vi "updater.vi"() -> ()   [LabVIEW 2014]
uses:
  <vilib>/Utility/sysdir.llb/System Directory Type.ctl
  subVI/version.vi
  <vilib>/Utility/config.llb/Read Key (String).vi
  <vilib>/FTP/NI_FTP.lvlib
  <vilib>/Utility/config.llb/NI_LVConfig.lvlib
panel:
  out "슬라이드":u8(slide) scale=1.0..3.0
  out "정보출력":string="업데이트 정보를 확인합니다."
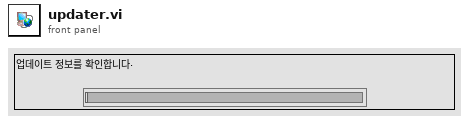
[diagram p1: front panel]
types:
  T1 = typedef "NI_FTP.lvlib/FTP Session.ctl" = refnum<k5>
  T2 = typedef "System Directory Type.ctl" = i32
  T3 = typedef "NI_LVConfig.lvlib/Config Data RefNum.ctl" = refnum<k1>
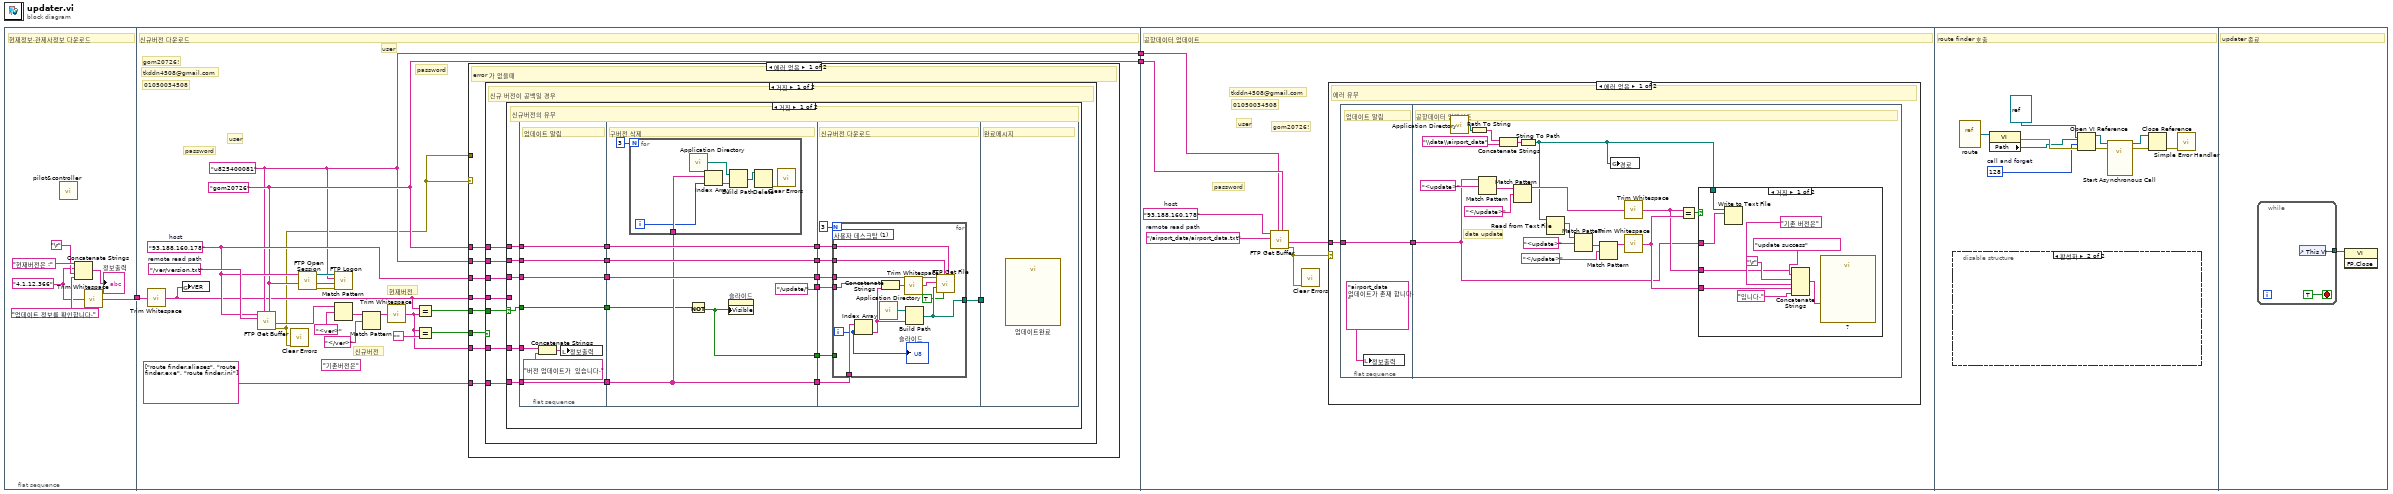
[diagram p0: block diagram]
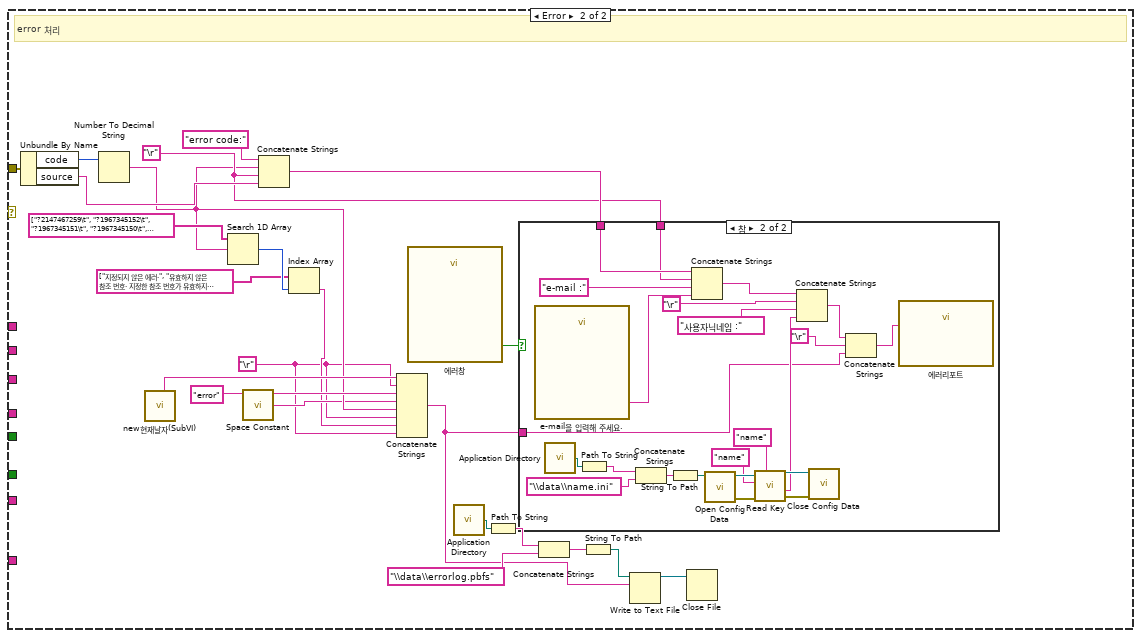
[diagram p4: hidden frame]
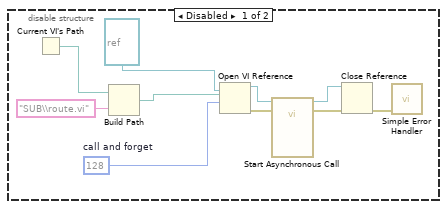
[diagram p8: hidden frame]
diagram:
  n1 = flat-sequence {
    tunnel: [w5] -> w1
    tunnel: [w17] -> w3
    tunnel: [w18] -> w2
    tunnel: w1 -> [w16]
    tunnel: w3 -> [w151]
    tunnel: w2 -> [w152]
    frame #0 {
      w4 = "4.1.12.366"
      # "현재정보,관제사정보 다운로드"
      n2 = call "pilot&controller.vi"() -> ()  [unwired: 11 in, 1 out]
      n3 = Concatenate Strings("현재버전은 :", w4, "\r", "업데이트 정보를 확인합니다." ("정보출력")) -> (→"정보출력":string)
      n4 = call <vilib>:"Trim Whitespace.vi"("string"=w4) -> ("trimmed string"=w5:string)  [unwired: 1 in]
    }
    frame #1 {
      (unwired) "기존버전은" ("문자열")
      w18 = "gom20726"
      w17 = "u825400081"
      w26 = "/ver/version.txt"  # remote read path
      w19 = "93.188.160.178"  # host
      # "신규버전"
      # "현재버전"
      # "password"
      # "user"
      # "gom20726!"
      # "01050034508"
      # "tkddn4508@gmail.com"
      # "user"
      # "password"
      # "신규버전 다운로드"
      n5 = call <vilib>:"Trim Whitespace.vi"("string"=w16) -> ("trimmed string"=w13:string)  [unwired: 1 in]
      n6 = global write "version.vi" "VER"(w13) -> ()
      n7 = call <vilib>:"FTP Get Buffer.vi"("password"=w18, "user"=w17, "remote path"=w26, "host"=w19) -> ("error out"=w12:errorcluster, "data"=w24:string)  [unwired: 5 in, 1 out]
      n8 = call <vilib>:"Clear Errors.vi"("error in (no error)"=w12) -> ()  [unwired: 5 in, 2 out]
      n9 = call <vilib>:"FTP Open Session.vi"("address"=w19) -> ("error out"=w28:errorcluster, "ftp session"=w27:T1)  [unwired: 7 in, 2 out]
      n10 = call <vilib>:"FTP Logon.vi"("error in (no error)"=w28, "password"=w18, "user"=w17, "ftp session"=w27) -> ()  [unwired: 4 in, 4 out]
      n11 = Match Pattern(string=w24, regular expression="<ver>" ("정규식")) -> (after substring=w23:string)  [unwired: 1 in, 3 out]
      n12 = Match Pattern(string=w23, regular expression="</ver>" ("정규식")) -> (before substring=w21:string)  [unwired: 1 in, 3 out]
      n13 = call <vilib>:"Trim Whitespace.vi"("string"=w21) -> ("trimmed string"=w14:string)  [unwired: 1 in]
      n14 = Equal?(x=w13, y=w14) -> (x = y?=w10:bool)
      n15 = Equal?(x=w14, y="") -> (x = y?=w11:bool)
      n16 = case shown="에러 없음" w12 {
        tunnel: w19 -> [w36 _]
        tunnel: w17 -> [w35 _]
        tunnel: w18 -> [w34 _]
        tunnel: string[] ["route finder.aliases", "route finder.exe", "route finder.ini"] -> [w33 _]
        tunnel: w12 -> [_ w125]
        tunnel: w13 -> [w32 _]
        tunnel: w14 -> [w31 _]
        tunnel: w11 -> [w30 _]
        tunnel: w10 -> [w29 _]
        frame No Error {
          # "error 가 없을때"
          n17 = case shown="거짓" w30 {
            tunnel: w36 -> [w43 _]
            tunnel: w35 -> [w42 _]
            tunnel: w34 -> [w41 _]
            tunnel: w33 -> [w40 _]
            tunnel: w32 -> [w39 _]
            tunnel: w31 -> [w38 _]
            tunnel: w29 -> [w37 _]
            frame False {
              # "신규 버전이 공백일 경우"
              n18 = case shown="거짓" w37 {
                selector: w37 -> [w45 _]
                tunnel: w43 -> [w61 _]
                tunnel: w42 -> [w60 _]
                tunnel: w41 -> [w59 _]
                tunnel: w40 -> [w58 _]
                tunnel: w39 -> [_ _]
                tunnel: w38 -> [w47 _]
                frame False {
                  # "신규버전의 유무"
                  n19 = flat-sequence {
                    tunnel: w58 -> [w66]
                    tunnel: w59 -> [w67]
                    tunnel: w60 -> [w68]
                    tunnel: w61 -> [w69]
                    tunnel: [w69] -> w51
                    tunnel: [w68] -> w50
                    tunnel: [w67] -> w49
                    tunnel: [w66] -> w48
                    tunnel: w47 -> [w63]
                    tunnel: [w62] -> w46
                    tunnel: w45 -> [w62]
                    tunnel: [w77] -> w57
                    tunnel: [w76] -> w56
                    tunnel: [w75] -> w55
                    tunnel: ["/update/" ("remote path")] -> w54
                    tunnel: [w73] -> w53
                    tunnel: w51 -> [w77]
                    tunnel: w50 -> [w76]
                    tunnel: w49 -> [w75]
                    tunnel: w48 -> [w73]
                    tunnel: w46 -> [w71]
                    tunnel: [w70] -> w44
                    tunnel: w57 -> [w91]
                    tunnel: w56 -> [w90]
                    tunnel: w55 -> [w89]
                    tunnel: w54 -> [w88]
                    tunnel: w53 -> [w86]
                    tunnel: [w85] -> w52
                    tunnel: w44 -> [w84]
                    tunnel: w52 -> [_]
                    frame #0 {
                      # "업데이트 알림"
                      n20 = Concatenate Strings(w63, "버전 업데이트가  있습니다." ("문자열")) -> (w65:string)
                      n21 = local write "정보출력"(w65) -> ()
                    }
                    frame #1 {
                      # "구버전 삭제"
                      n22 = for {
                        N: 3 -> [_]
                        tunnel: w73 -> [w79]
                        i -> [w78]
                        n23 = call <vilib>:"Application Directory.vi"() -> ("Application Directory"=w83:path)
                        n24 = Index Array(array=w79, index=w78) -> (element=w82:string)
                        n25 = Build Path(base path=w83, name or relative path=w82) -> (appended path=w81:path)
                        n26 = Delete(path (use dialog)=w81) -> (error out=w80:errorcluster)  [unwired: 4 in, 2 out]
                        n27 = call <vilib>:"Clear Errors.vi"("error in (no error)"=w80) -> ()  [unwired: 5 in, 2 out]
                      }
                      n28 = Not(x=w71) -> (.not. x?=w70:bool)
                      n29 = property on="슬라이드" class="Slide (엄격한)"("Visible"=w70) -> ()  [unwired: 2 in, 2 out]
                    }
                    frame #2 {
                      # "신규버전 다운로드"
                      n30 = for {
                        N: 3 -> [_]
                        tunnel: w91 -> [w103]
                        tunnel: w90 -> [w102]
                        tunnel: w89 -> [w101]
                        tunnel: w88 -> [w100]
                        tunnel: w86 -> [w97]
                        tunnel: [w96] -> w85
                        tunnel: w84 -> [_]
                        i -> [w92]
                        (unwired) T2 1 items=["사용자 홈"=0, "사용자 데스크탑"=1, "사용자 문서"=2, "사용자 어플리케이션 데이터"=3, "사용자 환경"=4, "사용자 임시"=5, "퍼블릭 문서"=6, "퍼블릭 어플리케이션 데이터"=7, "퍼블릭 환경"=8, "퍼블릭 캐시"=13, "시스템 코어 라이브러리"=9, "시스템 설치된 라이브러리"=10, "어플리케이션 파일"=11, "부팅 볼륨 루트"=12] ("system directory type")
                        n31 = Index Array(array=w97, index=w92) -> (element=w95:string)
                        n32 = call <vilib>:"Application Directory.vi"() -> ("Application Directory"=w93:path)
                        n33 = Concatenate Strings(w100, w95) -> (w99:string)
                        n34 = call <vilib>:"Trim Whitespace.vi"("string"=w99) -> ("trimmed string"=w98:string)  [unwired: 1 in]
                        n35 = Build Path(base path=w93, name or relative path=w95) -> (appended path=w96:path)
                        n36 = call <vilib>:"FTP Get File.vi"("password"=w101, "binary (F)"=TRUE, "user"=w102, "local path"=w96, "remote path"=w98, "host"=w103) -> ()  [unwired: 4 in, 2 out]
                        "슬라이드" <- w92
                      }
                    }
                    frame #3 {
                      # "완료메시지"
                      n37 = call "업데이트완료"() -> ()  [unwired: 10 in, 2 out]
                    }
                  }
                }
                frame True {
                }
              }
            }
            frame True {
            }
          }
        }
        frame Error {
          w105 = "\r"
          w120 = "\r"
          # "error 처리"
          n38 = Unbundle By Name(w125) -> ("code"=w124:i32, "source"=w122:string)
          n39 = Number To Decimal String(number=w124) -> (decimal integer string=w108:string)  [unwired: 1 in]
          n40 = call "new현재날자(SubVI).vi"() -> ("날짜/시간 문자열"=w110:string)  [unwired: 5 in, 6 out]
          n41 = Search 1D Array(1D array=string[] ["?2147467259\t", "?1967345152\t", "?1967345151\t", "?1967345150\t", "?1967345149\t", "?1967345148\t", "?1967345147\t", "?375012\t", "?375011\t", "?375010\t", "?375009\t", "?375008\t", "?375007\t", "?375005\t", "?375004\t", "?375003\t", "?375002\t", "?375001\t", "?375000\t", "?120000", "?4850\t", "?4824\t", "?4820\t", "?4803\t", "?4407\t", "?4406\t", "?4404\t", "?4403\t", "?4402\t", "?4401\t", "?4400\t", "?2584\t", "?2580\t", "1\t", "2\t", "4\t", "5\t", "6\t", "7\t", "8\t", "9\t", "10\t", "11\t", "12\t", "13\t", "14\t", "15\t", "16\t", "17\t", "18\t", "19\t", "20\t", "21\t", "22\t", "23\t", "24\t", "25\t", "26\t", "27\t", "28", "29\t", "30\t", "31\t", "32\t", "33\t", "34\t", "35\t", "36\t", "37\t", "38\t", "39\t", "40\t", "41\t", "42\t", "43\t", "44\t", "45\t", "46\t", "47\t", "48\t", "49\t", "50\t", "51", "52\t", "67\t", "68\t", "69\t", "70\t", "71\t", "72\t", "73\t", "74\t", "75\t", "81\t", "82\t", "83\t", "84\t", "85\t", "87\t", "88\t", "89\t", "90\t", "91\t", "97\t", "98\t", "99\t", "100\t", "116\t", "117\t", "118\t", "122\t", "123\t", "124\t", "125\t", "1000\t", "1001\t", "1002\t", "1003\t", "1004\t", "1005\t", "1006\t", "1007\t", "1008\t", "1009\t", "1010\t", "1011\t", "1012\t", "1013\t", "1014\t", "1015\t", "1016\t", "1017\t", "1018\t", "1019\t", "1022\t", "1023\t", "1024\t", "1025\t", "1026\t", "1027\t", "1028\t", "1029\t", "1030\t", "1031\t", "1032\t", "1033\t", "1034\t", "1035\t", "1036\t", "1037\t", "1038", "1039\t", "1040\t", "1041\t", "1042\t", "1043\t", "1044\t", "1045\t", "1051\t", "1052\t", "1054\t", "1055\t", "1056\t", "1057\t", "1058\t", "1059\t", "1060\t", "1061", "1062\t", "1063\t", "1066\t", "1067\t", "1068\t", "1069\t", "1070\t", "1071\t", "1072\t", "1073\t", "1074\t", "1075\t", "1076\t", "1077\t", "1082\t", "1086\t", "1087\t", "1088\t", "1089\t", "1090\t", "1091\t", "1094\t", "1095\t", "1096\t", "1097\t", "1098\t", "1100\t", "1102\t", "1103\t", "1104\t", "1105\t", "1106\t", "1107\t", "1108\t", "1109\t", "1110\t", "1111\t", "1122\t", "1123\t", "1124\t", "1125\t", "1126\t", "1127\t", "1128\t", "1129\t", "1130\t", "1131\t", "1135\t", "1136\t", "1137\t", "1138\t", "1144\t", "1145\t", "1146\t", "1147\t", "1148\t", "1149\t", "1150\t", "1151\t", "1156\t", "1157\t", "1174\t", "1175\t", "1176\t", "1177\t", "1186\t", "1187\t", "1188\t", "1190\t", "1191\t", "1192\t", "1193\t", "1194\t", "1196\t", "1197\t", "1198\t", "1301\t", "1303\t", "1304\t", "1305\t", "1306\t", "1307\t", "1308\t", "1309\t", "1310\t", "1311\t", "1312\t", "1313\t", "1314\t", "1315\t", "1319\t", "1320\t", "1321\t", "1322\t", "1357\t", "1358\t", "1359\t", "1360\t", "1361\t", "1362\t", "1363\t", "1364\t", "1365\t", "1366\t", "1370\t", "1376\t", "1377\t", "1378\t", "1380\t", "1381\t", "1384\t", "1385\t", "1388\t", "1389\t", "1390\t", "1396\t", "1397\t", "1398\t", "1399\t", "1430\t", "1432\t", "1434\t", "1436\t", "1438\t", "1439", "1440\t", "1443", "1444", "1445\t", "1447\t", "1449\t", "1450\t", "1451\t", "1452\t", "1453\t", "1454\t", "1455\t", "1468\t", "1469\t", "1470\t", "1483\t", "1484\t", "1485\t", "1488\t", "1489\t", "1490\t", "1491\t", "1492\t", "1493\t", "1497\t", "1498\t", "1499\t", "1500\t", "1502\t", "1503\t", "1504\t", "1517\t", "1523\t", "1524\t", "1526\t", "1529\t", "1532\t", "1533\t", "1534\t", "1535\t", "1544\t", "1545\t", "1546\t", "1548\t", "1550\t", "1553\t", "1554\t", "1556\t", "1557\t", "1558\t", "1564\t", "1571\t", "1573\t", "1574\t", "1579\t", "1580\t", "1581\t", "1584\t", "1586\t", "1587\t", "1588\t", "1590\t", "1595\t", "1596\t", "1597\t", "1599\t", "1603\t", "1604\t", "1611\t", "1616\t", "1617\t", "1619\t", "1620\t", "1621\t", "1622\t", "1623\t", "1624\t", "1627\t", "1628\t", "1629\t", "1630\t", "1632\t", "4800\t", "4801\t", "4802\t", "4803\t", "4804\t", "4805\t", "4806\t", "4810\t", "4811\t", "4820\t", "4821\t", "4822\t", "4823\t", "56000\t", "56001\t", "56002\t", "56003\t", "56004", "56005\t", "56006\t", "66464"] ("String Data"), element=w108) -> (index of element=w113:i32)  [unwired: 1 in]
          n42 = call <vilib>:"Space Constant.vi"() -> ("String"=w107:string)
          n43 = Concatenate Strings("error code:" ("문자열"), w108, w120, w122) -> (w121:string)
          n44 = Index Array(array=string[] ["지정되지 않은 에러.", "유효하지 않은 참조 번호. 지정한 참조 번호가 유효하지 않습니다.", "유효하지 않은 프로퍼티 코드. 지정한 프로퍼티 코드가 이 참조 번호에는 유효하지 않습니다.", "유효하지 않은 특권 ID. 지정한 특권 ID가 범위를 벗어납니다.", "유효하지 않은 접근 타입. 지정한 접근 타입이 유효하지 않습니다.", "유효하지 않은 인수. 지정한 인수 중 하나가 유효하지 않습니다.", "발견되지 않은 입력. 요청하신 입력을 찾을 수 없습니다.", "JSON 숫자값이 LabVIEW 숫자형 타입의 범위를 벗어납니다.", "LabVIEW가 무한대 또는 무한대 부동소수 값을 읽거나 쓰는데 실패했습니다. 무한대 값에 대한 지원을 허용하려면 LabVIEW JSON을 활성화해야 합니다.", "LabVIEW가 NaN 부동소수 값을 읽거나 쓰는데 실패했습니다. NaN 값에 대한 지원을 허용하려면 LabVIEW JSON을 활성화해야 합니다.", "JSON 문자열이 유효하지 않은 다차원 배열을 포함합니다.", "배열에 유효하지 않은 차원 수가 있습니다.", "클러스터 또는 JSON 문자열이 유효하지 않은 수의 원소를 포함합니다. 엄격한 검증이 활성화된 경우, JSON 문자열의 원소 개수는 입력 클러스터의 원소 개수와 반드시 일치해야 합니다.", "?375005\tJSON과 LabVIEW 간의 타입 불일치.", "JSON 문자열에서 경로를 찾을 수 없습니다.", "JSON 문자열이 유효하지 않습니다. JSON 문자열은 UTF-8로 인코딩되고, JSON 문법을 따라야 합니다.", "클러스터 원소 이름이 유효하지 않습니다. 클러스터의 각 원소는 고유한 이름을 가지거나, 빈 문자열의 경우와 같이 이름이 없어야 합니다.", "JSON 루트 컨테이너는 반드시 배열 또는 클러스터이어야 합니다.", "데이터 타입이 JSON으로 또는 JSON으로부터 변환될 수 없습니다. 지원되는 데이터 타입은 불리언, 숫자형, 문자열의 배열과 클러스터 및 기타 배열과 클러스터를 포함합니다.", "이 익스프레스 VI를 열려면 SignalExpress가 필요합니다. SignalExpress를 설치하거나 www.ni.com/signalexpress에서 평가판을 다운로드하십시오.", "디바이스 드라이버가 존재하지 않거나 지원하지 않습니다. 입력 포트와 출력 포트 VI를 실행하는데 필요한 디바이스 드라이버가 없습니다. LabVIEW는 Windows Vista 또는 이후 버전에서 이 디바이스를 지원하지 않습니다.", "[-1.0, 1.0] 범위를 맞추기 위해 잘려진 부동소수 데이터. 부동소수 데이터가 [-1.0, 1.0] 범위의 밖에 있었습니다. 값은 이 범위 안에 맞도록 잘렸습니다.", "버퍼 언더플로우가 발생하였습니다. 어플리케이션이 데이터를 쓰는 속도가 빠르지 않아 버퍼 언더플로우가 발생하였습니다.", "사운드 드라이버 또는 카드가 지정한 작업을 지원하지 않습니다. 사운드 드라이버 또는 카드가 지정된 설정과 호환되지 않습니다. 파라미터 값이 하드웨어 및 드라이버의 지원 범위 내에 있는지 확인합니다.", "LabVIEW가 팔레트 아이템을 찾을 수 없습니다. LabVIEW가 팔레트 아이템을 찾을 수 없습니다. 아이템 배열에 있는 각 아이템의 경로를 확인하십시오. 파일이 이동 또는 삭제되었거나, 경로가 OS에 맞지 않게 포맷되었을 수 있습니다. 예를 들면, 경로 분리자로서 Windows에서는 \\, OS X(32비트)에서는 :, Linux와 OS X(64비트)에서는 /를 사용합니다.", "이 LabVIEW 버전에서 지원하지 않는 VI 아이템이 팔레트 데이터 배열에 있습니다. 이 LabVIEW 버전에서 지원하지 않는 VI 아이템이 팔레트 데이터 배열에 있습니다. 이 에러는 LabVIEW 런타임 엔진에서 지원되지 않는 VI를 사용하는 경우에 발생할 수 있습니다.", "팔레트 폭에 대한 값이 유효하지 않습니다. 팔레트 폭의 값은 0보다 크거나 같아야 합니다.", "유효하지 않은 팔레트 아이템이 있습니다. 유효하지 않은 팔레트 아이템이 있습니다. 아이템 배열에 있는 각 아이템의 경로를 확인하십시오. VI와 팔레트 파일(.mnu)에 대한 경로가 유효해야 합니다.", "팔레트 보기 포맷이 유효하지 않습니다. 팔레트 보기 포맷은 아이콘, 아이콘과 텍스트, 또는 텍스트가 되어야 합니다. 컨트롤 또는 함수 팔레트에서 사용자 정의≫이 팔레트 보기를 선택하여 팔레트 보기 포맷을 변경합니다.", "지정한 파일이 유효한 팔레트 파일(.mnu)이 아닙니다. 지정한 파일이 유효한 팔레트 파일(.mnu)이 아닙니다. 기존 팔레트 파일에 대한 경로를 입력하여 팔레트 파일로부터 데이터를 읽습니다. 유효한 팔레트 파일에 대한 경로를 입력하여 파일에 데이터를 씁니다.", "팔레트 타입이 유효하지 않습니다. 팔레트 타입 입력이 유효하지 않습니다. 팔레트 타입 값이 컨트롤 또는 함수의 열거형 값을 갖고 있습니다. 제공한 값이 정의된 범위를 벗어났습니다.", "DIAdem을 시작할 수 없습니다. DIAdem 리포트 익스프레스 VI를 사용하려면 반드시 DIAdem 9.1 Service Pack 2나 이후 버전이 설치되어 있어야 합니다.", "[측정 파일에 쓰기] 익스프레스 VI는 새로운 데이터를 주파수 영역 웨이브폼에 추가할 수 없습니다. 주파수 영역 웨이브폼은 기본 주파수 f0 와 델타 주파수 df 로 구성되어 있습니다. 그러므로, 데이터 포인트의 주파수는 f0+N*df 로 계산됩니다. 이 계산은 데이터가 웨이브폼에 추가된 경우에는 많은 에러를 유발합니다. 부분 헤더를 하나의 헤더만으로 설정한 후 주파수 영역 웨이브폼을 파일에 쓸 때 이 에러가 발생할 수 있습니다. 부분 헤더를 부분마다 하나의 헤더로 설정하여 이 에러를 수정합니다.", "입력 파라미터가 유효하지 않습니다. 예를 들어 입력이 경로이면 경로에는 ? 또는 @와 같이 OS에 의해 허용되지 않은 문자가 있을 수 있습니다. 파일 I/O VI를 실행하려고 시도하는 동안 이 에러가 발생했다면, 더 자세한 정보는 ni.com에서 기술지원 데이터베이스를 참조하십시오.", "메모리가 꽉 찼습니다 큰 어플리케이션을 개발하거나 LabVIEW에서 큰 데이터 세트를 저장하는 동안 이 에러가 발생했다면, 더 자세한 정보는 ni.com에서 기술지원 데이터베이스를 참조하십시오.", "파일 끝입니다.", "파일이 이미 열려 있습니다.", "일반 파일 I/O 에러. 이 에러의 가능한 원인은 저장하려는 디스크나 하드 드라이브가 꽉 찼다는 것입니다. 디스크 공간을 비우거나 다른 디스크나 드라이브에 저장하십시오. 네트워크 연결이 좋지 않아서 이 에러가 발생할 수 있습니다. 예를 들어, 네트워크 연결이 끊겼거나 네트워크 케이블이 꽂혀있지 않을 수도 있습니다.", "파일을 찾을 수 없습니다. 파일이 다른 위치에 있거나 삭제되었습니다. 명령 입력요청이나 파일 탐색기를 사용하여 경로가 올바른지 확인합니다. 네트워크 연결이 좋지 않아서 이 에러가 발생할 수 있습니다. 예를 들어, 네트워크 연결이 끊겼거나 네트워크 케이블이 꽂혀있지 않을 수도 있습니다.", "파일 권한 에러. 파일에 대해 올바른 권한이 없습니다. 에러를 수정하려면 다른 어플리케이션이 파일을 사용하고 있지 않으며 파일 권한이 바르게 설정되었는지 확인하십시오. Windows의 경우, 파일을 탐색하고, 파일에서 마우스 오른쪽 버튼을 클릭한 다음, 프로퍼티를 선택하고 대화 상자에서 읽기 전용 옵션을 설정하십시오. Linux 또는 Mac OS X의 경우, chmod를 사용하여 파일 권한을 설정하십시오. 읽기 접근만 필요하다면, 접근 입력이 읽기 전용으로 설정된 상태에서 [파일 열기/생성/대체] 함수를 사용할 수 있습니다. Report Generation toolkit 1.1.2 또는 이후 버전을 사용하여 LabVIEW 8.5 또는 이후 버전의 실행 파일을 만드려고 시도하는 동안 이 에러가 발생했다면, 더 자세한 정보는 ni.com에서 기술지원 데이터베이스를 참조하십시오.", "디스크가 꽉참. 디스크 또는 하드 드라이브는 작업을 완료하는데 충분한 공간을 가지고 있지 않습니다. 디스크 공간을 비우거나 다른 디스크나 드라이브에 저장하십시오.", "복사된 경로. LabVIEW에서 어플리케이션을 빌드하는 동안 이 에러가 발생했다면, 더 자세한 정보는 ni.com에서 기술지원 데이터베이스를 참조하십시오. 파일 I/O 또는 VI를 사용하는 동안 이 에러가 발생했다면, 기존 파일 또는 폴더를 덮어 쓰려고 시도하는 중일 수 있습니다. 파일 또는 폴더 덮어쓰기에 대한 더 자세한 정보는 LabVIEW 도움말에서 특정 함수 또는 VI에 대한 참조 토픽을 참조하십시오.", "너무 많은 파일이 열려 있습니다.", "작동을 위해 필요한 일부 시스템 용량이 활성화되어 있지 않습니다.", "찾을 수 없는 외부 기호나 의존성 때문에 또는 유효하지 않은 파일 포맷 때문에 다이나믹 라이브러리를 로드하는데 실패했습니다.", "리소스 추가 불가.", "리소스를 찾을 수 없습니다. 이 에러는 독립 어플리케이션을 만들 때 VI의 프런트패널을 삭제한 경우 발생할 수 있습니다.", "이미지를 찾을 수 없습니다.", "이미지를 다루기 위한 메모리가 충분하지 않습니다.", "펜은 존재하지 않습니다.", "설정 타입이 유효하지 않습니다.", "토큰 설정을 찾을 수 없습니다.", "설정 문자열을 분석할 때 발생한 에러.", "메모리 설정 에러.", "적절치 않은 외부 코드 포맷.", "외부 서브루틴이 지원되지 않습니다.", "외부 코드가 없습니다.", "널 윈도우.", "윈도우 에러 제거.", "널 메뉴. 탈착 가능한 디바이스를 다시 연결한 경우, 이 디바이스를 다시 사용하려면 LabVIEW를 다시 시작해야할 수도 있습니다.", "인쇄 강제 종료.", "적절치 않은 인쇄 레코드.", "인쇄 드라이버 에러.", "인쇄하는 동안 발생하는 OS 에러.", "인쇄 중 메모리 에러.", "인쇄 대화 상자 에러.", "일반 인쇄 에러.", "유효하지 않은 디바이스 참조 번호.", "디바이스를 찾을 수 없습니다.", "디바이스 파라미터 에러.", "디바이스 단위 에러.", "디바이스 열기 불가.", "디바이스 호출 강제 종료.", "일반 에러.", "사용자에 의해 작업이 취소되었습니다. 이 에러가 발생한 VI 또는 함수가 에러 출력 파라미터를 갖는 경우, 에러 출력을 케이스 구조의 선택자 터미널에 연결하여 이 에러 메시지가 생기지 않도록 방지합니다. [파일 열기/생성/대체] 함수 또는 [데이터로그 열기/생성/대체] 함수를 사용하는 경우, 대신에 취소됨을 케이스 구조의 선택자 터미널에 연결할 수 있습니다. VI 또는 함수가 에러 출력을 갖고 있지 않은 경우, VI 또는 함수 내의 에러 핸들링을 편집하여 이 에러를 방지할 수 있습니다. VI 또는 함수에서 더블 클릭하고, 일반 에러 핸들링을 에러 출력 인디케이터 또는 다른 형식의 에러 핸들링으로 대체합니다. 새 VI 또는 함수를 vi.lib가 아닌 다른 디렉토리에 저장하여, 원본을 덮어쓰지 않도록 주의합니다.", "객체 ID 가 너무 낮습니다.", "객체 ID 가 너무 높습니다.", "객체가 히프에 없습니다.", "알수없는 히프.", "알수없는 객체 (유효하지 않은 DefProc).", "알수없는 객체 (DefProc 가 테이블에 없습니다).", "메시지가 범위를 벗어납니다.", "널 메소드.", "알 수 없는 메시지.", "인터어플리케이션 관리자 초기화 에러.", "적절치 않은 어커런스.", "핸들러가 어떤 어커런스를 기다려야 할 것인지 알지 못합니다.", "어커런스 큐 오버플로우.", "파일 데이터로그 타입 충돌.", "세마포어 신호가 없음.", "인터어플리케이션 관리자가 알아차리지 못하는 타입 에러.", "메모리나 데이터 구조 충돌.", "임시 DLL 만들기 실패.", "포맷 지정자 타입이 일치하지 않습니다. 포맷 지정자가 [문자열로 포맷]이나 [문자열로부터 스캔] 함수에 상응하는 인수에 데이터 타입과 일치하지 않습니다.", "알 수 없는 포맷 지정자. 적절하지 못한 포맷 지정자가 [문자열로 포맷]이나 [문자열로부터 스캔] 함수로의 포맷 문자열에서 발견되었습니다.", "너무 적은 포맷 지정자. [문자열로 포맷]이나 [문자열로부터 스캔] 함수의 모든 인수와 일치하는 포맷 지정자가 충분하지 않습니다.", "너무 많은 포맷 지정자. [문자열로 포맷]이나 [문자열로부터 스캔] 함수의 인수의 개수보다 더 많은 포맷 지정자가 있습니다.", "스캔을 실패하였습니다 입력 문자열이 예상된 포맷으로 데이터를 가지고 있지 않습니다. [문자열로부터 스캔] 함수는 그 입력을 스캔할 수 없었는데, 왜냐하면 데이터가 기대했던 포맷이 아니었기 때문입니다. [문자열로부터 스캔] 함수에서 마우스 오른쪽 버튼을 클릭하고t 포맷 문자열 편집을 선택하여 입력 데이터에 맞는 포맷 문자열을 설정하십시오. 또한 파일로부터 스캔 또는 문자열로부터 스캔 함수가 파일의 끝에 도달할 경우, 이 에러가 발생할 수 있습니다. 이러한 사용의 경우에 대한 더 자세한 정보는 ni.com의 기술지원 데이터베이스를 참조하십시오.", "배리언트로 변환 에러. LabVIEW 타입에서 OLE 배리언트 타입으로 변환하는데 발생한 에러입니다.", "런타임 메뉴 에러.", "다른 사용자에 의해 VI 암호가 바뀌었다.(@@)", "배리언트 속성을 찾을 수 없습니다.", "배리언트의 데이터 타입이 타입 입력에 연결된 데이터 타입과 호환하지 않습니다.", "널 또는 이미 삭제된 참조 번호가 입력으로 전달되었습니다.", "맞지 않는 파일 타입. 작동과 호환되지 않는 타입의 파일로부터 읽으려고 시도하거나 파일로 쓰려고 시도했습니다. 이 파일은 일반적으로 사용자 데이터 파일입니다.", "맞지 않는 파일 버전. 쓰거나 읽는 함수 버전과 호환되지 않는 버전의 파일로부터 읽거나 그 파일에 쓰려고 시도했습니다. 이 파일은 일반적으로 사용자 데이터 파일입니다.", "파일은 잘못된 데이터를 가지고 있습니다. 이 파일은 일반적으로 사용자 데이터 파일입니다.", "충돌이 일어나거나, 예상치 못하거나, 잘려나간 데이터때문에 패턴화 해제나 바이트 스트림 읽기 동작이 실패했습니다.", "파일 경로가 요구되는 곳에 디렉토리 경로를 제공했습니다. 파일 이름을 가진 파일 경로가 필요하나, 제공된 경로는 디렉토리에 대한 경로입니다.", "제공된 폴더 경로가 존재하지 않습니다.", "열고자 하는 리소스가 좀 더 최신 버전의 LabVIEW에서 생성되어 이 버전과 호환되지 않습니다.", "타임아웃이 발생했습니다.", "문자열에 예상하지 않은 널 문자가 포함되어 있습니다.", "스택 오버플로우가 발생했습니다. 이 에러를 수정하려면, LabVIEW를 다시 시작해서 재귀 데이터 구조가 없는지 코드를 검토하십시오.", "VI가 이 작업에 호환되는 상태에 있지 않습니다. 여러 이유로 인해 이 에러가 발생할 수 있습니다. 실행 중이거나 실행하려고 예약된 VI를 편집하려고 시도할 때 이 에러가 발생할 수 있습니다. 실행 중이거나 실행하려고 예약된 VI에 대한 참조를 열려고 시도할 때 이 에러가 발생할 수 있습니다. [VI 참조 열기] 함수에 타입 지정자 VI 참조 번호를 연결하여 VI에 대한 참조를 열 때, 또는 실행 VI 안에서 VI에 링크된 [정적 VI 참조]를 가질 때 VI는 실행이 예약됩니다. 또한 타겟 VI가 실행 중에 있거나 실행하려고 예정되어 있는 동안 VI를 실행하는 경우, 이 에러가 발생할 수 있습니다. 이 에러를 수정하려면, 타겟 VI가 유휴 상태이거나 재호출이 가능한지 확인합니다. 재호출이 가능한 경우, 옵션입력을 0x08로 설정하여 VI 재호출 실행을 준비한 상태 혹은 엄격한 타입의 VI 참조에 타입 지정자 VI 참조 번호를 연결한 상태에서 [VI 참조 열기] 함수를 사용합니다. 또한 이 에러는 VI가 프로그램적으로 수정되는 동안 VI의 이미지를 얻으려고 시도할 때 발생할 수 있습니다. 패널이나 다이어그램의 이미지를 얻으려면 VI가 변경 중이 아닐 때까지 기다립니다.", "VI 프런트패널이 열려있지 않습니다. 윈도우 모양 페이지를 사용하여 VI가 실행 중이거나 로드된 상태에서 프런트패널이 보이는지 설정하십시오. 또한 프런트패널:열기 메소드를 사용하여 프로그램적으로 프런트패널 윈도우를 열 수 있습니다.", "VI가 에러 상태에서 프런트패널 컨트롤을 가지고 있기 때문에 이 VI는 실행할 수 없습니다.", "VI는 실행 가능하지 않습니다. 이 에러는 VI가 깨졌거나 LabVIEW가 찾을 수 없는 SubVI가 포함되어 있기 때문에 발생할 수 있습니다. 파일≫열기를 선택하여 이 VI를 열어 실행할 수 있는지 확인합니다. 다음 중 하나의 상황에서 이 에러가 발생했을 경우, ni.com에서 기술지원 데이터베이스를 참조하십시오: VI 서버를 사용하여 다이나믹하게 VI 호출하기 또는 어플리케이션 빌드하기.", "VI가 메모리에 없습니다.", "VI 실행이 VI 프로퍼티 대화 상자에서 비활성화되었습니다. VI 프로퍼티 대화 상자의 실행 페이지를 열고 VI 실행에 대한 셋팅을 변경하십시오.", "커넥터 팬에서 FPDCO는 상수라고 생각합니다.", "요약된 IP 기록이 없습니다.", "커넥터 팬을 로드할 수 없습니다.", "범위를 벗어나는 배리언트 태그.", "기본값이 없거나 데이터를 수행하지 않습니다.", "VI 생성이 실패했습니다.", "블록다이어그램을 로드할 수 없습니다.", "프런트패널을 로드할 수 없습니다. 독립 어플리케이션을 만들 때 VI의 프런트패널을 포함하도록 확인합니다.", "링크 에러.", "프린터가 응답하지 않습니다. 프린터 설정을 확인합니다.", "히스토리를 로드할 수 없습니다.", "VI를 최근에 로드하고 저장한 이 후 이 VI를 디스크에서 변경하지 않았습니다.", "지정되지 않은 에러가 발생했습니다.", "하나 혹은 그 이상의 제목없는 SubVI가 있습니다. 모든 종속 파일의 이름을 만들기 전에는 이 파일을 저장할 수 없습니다.", "마법사 템플릿을 찾을 수 없습니다.", "마법사 템플릿이 다이어그램을 가지고 있지 않습니다.", "인스트루먼트 호출이 강제 종료되었습니다.", "어플리케이션 참조가 유효하지 않습니다.", "VI 참조가 유효하지 않습니다.", "요청된 작업에서, 참조가 요청된데로 예약될 수 없거나, 적절치 못한 예약 모드이거나, 실행 상태가 실행중이거나 예약되었습니다.", "속성 선택자가 유효하지 않습니다.", "VI 서버 프로퍼티가 읽기 전용입니다.", "VI 참조는 이미 편집을 위해 예약되어 있습니다.", "VI 참조 타입이 VI 커넥터 팬과 일치하지 않습니다.", "VI 서버 접근이 거부되었습니다. 이 에러가 원격 연결 상태의 VI 참조 열기 함수에서 반환되었다면, 옵션 대화 상자의 VI 서버 페이지를 사용하여 VI가 반출되었는지 확인하십시오. 이 에러가 프로퍼티 또는 인보크 노드에서 반환되었다면, 프로퍼티나 메소드가 원격 VI 서버 연결이 허용되지 않았을 수도 있습니다. 예를 들어, 로컬에서 어플리케이션:메모리 상의 모든 VI 프로퍼티를 사용할 수 있지만, 대신 원격에서는 어플리케이션:메모리 상의 VI 반출 프로퍼티를 사용해야 합니다. 프로퍼티 또는 메소드 도움말을 참고하여 원격에서 사용 가능한지 확인하십시오.", "적절치 않은 런타임 메뉴 파일 버전.", "적절치 않은 런타임 메뉴 파일.", "수행이 VI의 이 타입에 대해 유효하지 않습니다.", "메소드 선택자가 유효하지 않습니다.", "호환될 수 없는 VI 서버 프로토콜 버전.", "요구된 파라미터를 찾을 수 없습니다.", "VI가 강제 종료되었습니다.", "VI는 암호로 보호되어 있습니다.", "맞지 않는 암호.", "재귀 호출을 시도했습니다.", "프로퍼티 혹은 메소드가 LabVIEW의 이 버전에서 지원되지 않습니다. 이 에러는 LabVIEW 런타임 엔진에서 지원되지 않는 프로퍼티 또는 메소드를 사용했을 경우 발생할 수 있습니다.", "VI가 잠겨 있습니다.", "참조 닫기에 전달된 널 참조 번호.", "이 이름의 LabVIEW 파일이 메모리에 이미 존재하거나 또는 메모리에 있는 프로젝트 라이브러리 내에 존재합니다. 이 에러를 해결하려면, 파일의 이름을 어플리케이션 인스턴스에 없는 유일한 이름으로 지정합니다.", "LabVIEW 파일 이름이 유효하지 않습니다.", "지정된 객체가 발견되지 않았습니다.", "객체 참조가 유효하지 않습니다.", "지정된 객체가 이 버전에서 쓰일 수 없습니다.", "타입 불일치: 객체가 지정된 타입으로 캐스트될 수 없습니다.", "지정된 프로퍼티를 찾을 수 없습니다.", "예상하지 않은 파일 타입.", "객체는 지정된 객체를 가질 수 없습니다.", "새로운 객체를 생성할 수 없습니다.", "지정된 객체들이 함께 연결될 수 없습니다.", "지정된 터미널이 객체에서 발견되지 않습니다.", "하드웨어 열기 에러.", "하드웨어 닫기 에러.", "하드웨어 수행 에러.", "하드웨어 DLL을 찾을 수 없음.", "하드웨어의 세션 에러가 없음.", "LabVIEW가 지정한 메소드를 찾을 수 없습니다.", "이 프로퍼티나 메소드가 아직 실행되지 않습니다.", "이 VI가 편집 모드에 있을 때만 이 프로퍼티를 쓸 수 있거나, 이 VI가 편집 모드에 있을 때만 이 메소드를 사용할 수 있습니다. 이 에러에 대한 추가적인 정보는 기술지원 데이터베이스를 참조하십시오.", "지정된 터미널에서 컨트롤/인디케이터를 생성할 수 없습니다.", "지정된 터미널에서 상수를 생성할 수 없습니다.", "VI는 디버깅할 수 없습니다.", "유효하지 않은 프로퍼티 값.", "엄격한 타입 정의 인스턴스에서 수행이 유효하지 않습니다.", "잘못된 컨트롤 타입. 이 종류의 컨트롤이나 이 레벨의 컨트롤에서 수행이 허용되지 않습니다.", "객체에 대해 사용할 수 있는 DataSocket 정보가 없습니다.", "파라미터에 대한 잘못된 값.", "스크립트를 실행하는 동안 발생한 에러. 서버로부터 에러 메시지: %s.", "지정된 객체를 움직일 수 없습니다.", "VI 서버나 클라이언트가 인식하지 못하는 메시지를 받았습니다.", "같은 이름의 큐와 알림자 참조는 같은 데이터 타입을 사용하여 얻어져야 합니다. 큐나 알림자에 대한 참조를 얻을 때, 어느 데이터 타입으로 이 메커니즘을 저장할지 지정할 수 있습니다. 동일한 메커니즘에 대한 참조를 얻기 위한 미래의 요청을 원래 지정한 데이터 타입과 같은 데이터 타입에 연결하지 않았을 때 이 에러가 발생할 수 있습니다. 이름 없는 메커니즘은 이러한 제한을 가지고 있지 않은데, 그 이유는 이름 없는 메커니즘을 얻으려는 각 요청이 새로운 메커니즘을 생성하기 때문입니다. 이 에러를 방지하는 것에 대한 더 자세한 정보는 ni.com의 기술지원 데이터베이스를 참조하십시오.", "이 컨테이너는 서브타입 없이 남겨질 수 없습니다. 컨테이너 경계에서 마우스 오른쪽 버튼을 클릭하고 대체를 선택하거나 새 서브타입을 끌어 옵니다.", "[VI 참조 열기] 함수는 재호출 실행을 위해 재호출되지 않는 VI를 준비할 수 없습니다. [VI 참조 열기] 함수에 연결한 값을 확인합니다.", "[라이브러리 함수 호출 노드]에 의해 호출된 외부 코드 안에서 예외가 발생했습니다. 이 같은 예외로 LabVIEW 메모리가 손상했을 수 있습니다. 새 위치에 모든 작업을 저장하고 LabVIEW를 다시 시작합니다. [라이브러리 함수 호출 노드]에 연결한 값을 확인합니다.", "블록다이어그램을 이용할 수 없다면 타입 정의나 다형성 VI로의 연결을 끊을 수 없습니다.", "해당 이름의 객체를 찾을 수 없었습니다. 어떤 참조도 반환될 수 없습니다. [큐 얻기] 함수나 [알림자 얻기] 함수를 사용하여 이름으로 큐나 알림자를 찾을 수 있습니다. 발견되지 않으면 생성?이 거짓이고 그 이름을 가진 큐나 알림자가 발견되지 않으면, LabVIEW는 이 에러를 반환합니다.", "xml 문자열 입력에 연결된 문자열이 비어 있습니다.", "데이터의 타입을 설명하는 XML 태그가 인식되어 있지 않습니다.", "XML 시작/끝 태그에 대해 끝 태그가 발견되지 않았습니다.", "알려져 있지 않거나 기대하지 않던 XML 태그가 발견되었습니다.", "데이터의 타입을 설명하는 XML 태그는 연결된 타입과 일치하지 않습니다.", "XML 열거형 타입 선택은 연결된 타입과 일치하지 않습니다.", "XML 값 텍스트는 적절하지 않거나 타입과 포맷을 위한 범위에서 벗어납니다.", "지원받지 않는 데이터 타입.", "더 이상 사용되지 않습니다.", "[세마포어 해제]가 현재 얻지 못한 세마포어를 호출했습니다.", "참조 번호는 노드가 그것을 기다리는 동안 유효하지 않게 되었습니다.", "빌드 어플리케이션에서 컨트롤 캡션과 같은 객체를 생성할 수 없습니다. LabVIEW 개발 시스템에서 이 객체를 생성해야 합니다.", "VI는 로드할 수 없습니다. 로드 중인 VI가 다른 OS에 대해 컴파일되었거나, SSE와 같이 타겟이 지원하지 않는 CPU 구성 요소와 함께 마지막으로 컴파일되었을 경우 빌드된 어플리케이션에서 이러한 에러가 일어날 수 있습니다. 이러한 경우에는 어플리케이션을 타겟 OS에 대해 다시 빌드하고 빌드 스펙의 SSE 컴파일러 셋팅이 타겟 플랫폼과 일치하도록 해야 합니다. 이 에러는 VI가 LabVIEW 런타임 엔진에서 로드될 수 없는 다형성 VI인 경우에 나타날 수 있습니다. 다형성 VI 자체가 아니라 다형성 VI의 인스턴스를 로드해야 합니다.", "파일 버전이 현재 LabVIEW 버전보다 더 나중의 것입니다.", "VI 버전이 너무 오래되어 현재 LabVIEW 버전으로 변환할 수 없습니다. 현재 LabVIEW 버전으로 VI를 변환하는 방법에 대한 추가적인 정보는 LabVIEW 도움말에서 VI 변환하기 토픽을 참조하십시오.", "템플릿 VI가 이미 메모리에 있으므로 그것을 예를 들어 설명할 수 없습니다.", "입력 단위가 현재 단위와 호환되지 않습니다.", "링 컨트롤에서 두 개 이상의 문자열에 같은 숫자형 값을 할당할 수 없습니다. 또한 콤보 박스 컨트롤에서 두 개 이상의 문자열에 같은 문자열 값을 할당할 수 없습니다. 컨트롤의 문자열과 값[] 프로퍼티에 쓰려고 시도하는 도중 이 에러가 발생했다면, 더 자세한 정보는 ni.com의 KnowledgeBase 를 참조하십시오.", "VI 서버의 연결 피어가 응답하지 않습니다. 연결 폴링에 대한 추가적인 정보는 LabVIEW 도움말의 연결 응답: 확인 메소드 토픽을 참조하십시오.", "이 시스템 컨트롤로 이 프로퍼티를 사용할 수 없습니다.", "트리 컨트롤의 활성화 아이템이 이 프로퍼티에서 유효하지 않습니다.", "유효하지 않은 아이템 태그를 트리 컨트롤 프로퍼티나 메소드에 연결했습니다.", "트리 컨트롤의 내적인 데이터가 손상되어 있습니다.", "LabVIEW가 호출한 외부 코드 내에서 예외가 발생했습니다. 이로 인해 LabVIEW 메모리가 손상했을 수 있습니다. 새 위치에 모든 작업을 저장하고 LabVIEW를 다시 시작합니다.", "VI가 이미 열려 있으므로 서브패널 컨트롤에 VI를 삽입할 수 없습니다.", "VI가 이미 서브패널 컨트롤에 있으므로 VI를 열 수 없습니다.", "하위 전용 아이템을 상위 아이템으로 변경하는 작업을 시도했습니다.", "서브패널 컨트롤에서 원격 VI를 삽입할 수 없습니다.", "이 프로퍼티는 VI가 서브패널에 있는 동안 읽기 전용입니다.", "닫힌 프런트패널의 상태를 닫거나 설정할 수 없습니다. 프런트패널을 닫거나 그 상태를 설정하기 전에 프런트패널이 이미 열려 있어야 합니다.", "이미 열려 있는 프런트패널을 열 수 없습니다. 열린 프런트패널의 상태를 설정하려면 프런트패널 윈도우:상태 프로퍼티를 사용합니다.", "프런트패널 상태에 대해 유효하지 않은 입력.", "데이터 포맷이 기대했던 데이터 타입과 일치하지 않아서 발생한 메모리에 꽉 참 에러. 이것은 메모리에 너무 큰 버퍼를 할당하려고 해서 생깁니다. 정상적인 메모리 할당도 시스템 메모리를 다 차지할 수 있지만, 메모리 부족 에러는 대부분 데이터를 잘못 해석하고 데이터를 데이터 크기로 처리하기 때문에 발생합니다. 시스템이 작업을 끝마치기 위해 더 많은 메모리를 필요로 한다고 가정하기 전에, 요청하는 읽기 포맷이 읽는 데이터에 유효한지 확인합니다.", "숫자형 인디케이터를 가지고 이 프로퍼티를 사용할 수 없습니다.", "[라이브러리 함수 호출 노드]에 대해 유효하지 않은 반환 파라미터. 반환 타입은 Void, 숫자형, 또는 문자열입니다. 숫자형 반환 타입은 값으로 전달됩니다. 문자열 반환 타입은 C 문자열 포인터나 Pascal 문자열 포인터로서 전달됩니다.", "[라이브러리 함수 호출 노드] 설정에서 유효하지 않은 배열 차원. 배열은 1차 이상의 차원을 가져야 합니다.", "[라이브러리 함수 호출 노드] 설정에서 유효하지 않은 웨이브폼 차원. 웨이브폼은 0 이나 1 차원을 가져야 합니다.", "라이브러리 함수 호출 노드 파라미터에 대해 유효하지 않은 데이터 타입. Void는 함수의 반환 타입으로만 사용될 수 있습니다.", "자체에 라벨을 보여 주거나 숨길 수 없습니다. 라벨을 보이는 것은 라벨 소유자가 컨트롤합니다.", "이 작업을 위해 Internet Explorer가 필요하지만 설치되어 있지 않습니다.", "정적 VI 참조가 설정되어 있지 않습니다. 블록다이어그램의 정적 VI 참조 함수에서 마우스 오른쪽 버튼을 클릭하고 경로 탐색을 선택합니다. 참조를 위해 VI를 탐색하고 참조를 설정하기 위해 열기 버튼을 클릭합니다.", "컨트롤이 키 포커스를 가질 때 수행이 허용되지 않습니다.", "와이어가 이미 그 위에 프로브를 가지고 있습니다.", "디지털 디스플레이를 위한 데이터 범위 설정이 없습니다.", "불리언 컨트롤이 래치 기계적인 동작을 할 때, 값 프로퍼티를 사용하여 값을 읽거나 쓸 수 없습니다. 불리언 컨트롤이 래치 기계적 동작으로 설정된 경우, 값 프로퍼티는 항상 에러를 반환합니다. 래치 기계적 동작으로 설정된 불리언 값이 있을 때 경합 조건이 발생할 수 있기 때문에 래치 기계적 동작으로 설정된 불리언 값을 프로그램적으로 읽을 수 없습니다.", "이 익스프레스 VI는 DIAdem 8.1 이상의 버전과 LabVIEW DIAdem 연결 VI 버전 2.1 이상을 요구합니다. 연결 VI는 ni.com에서 무료로 다운로드 받을 수 있습니다. 이 VI를 다운로드하려면 National Instruments 웹 사이트를 참조하십시오.", "확장 가능한 subVI의 확장된 영역에서 같은 터미널을 한번 이상 열거할 수 없습니다.", "이 작업은 정적 VI 참조에서 유효하지 않습니다. 정적 VI 참조를 사용하여 VI를 실행하려면, 인보크 노드를 사용하여 VI 실행 메소드를 호출합니다. VI에 인보크 노드 클래스를 설정하여 VI 실행 메소드를 선택합니다.", "VI가 이 작업에 호환되는 상태에 있지 않습니다. 참조된 VI의 실행 모드를 변경하여 이 작업을 재호출합니다.", "전달된 배열의 차원이 작업을 수행하는데 기대되었던 차원과 일치하지 않습니다.", "배열의 원소가 유일하지 않습니다. 배열에 중복된 아이템이 있습니다.", "배열 인덱스가 배열의 경계 밖에 있습니다.", "요구된 페이지를 발견할 수 없습니다.", "새로운 코드 리소스를 노드에 로드할 수 없습니다. 코드 리소스가 이미 로드되어 있습니다.", "서브패널 컨트롤이 VI 윈도우를 열 수 없습니다. 서브패널 컨트롤에 VI를 삽입하려고 했지만, 삽입하려는 프런트패널이나 블록다이어그램 윈도우가 존재하지 않습니다.", "프로퍼티나 인보크 노드가 프런트패널 컨트롤에 링크되어 있지 않습니다.", "프로퍼티나 인보크 노드 참조 입력 터미널이 이미 연결되어 있습니다.", "객체가 프로퍼티 또는 인보크 노드와 같은 VI에 있지 않습니다. 컨트롤의 컨트롤 참조가 프로퍼티나 인보크 노드를 가지고 있는 VI에 속해 있지 않습니다.", "클래스 이름에 대한 입력이 올바르지 않거나 틀린 포맷입니다. 클래스 이름에 대한 입력이 올바르지 않거나 틀린 포맷입니다. 올바른 포맷은 클래스 타입으로 시작하여 그 뒤에 긴 이름을 사용한 객체 경로가 와야 합니다. 예를 들면, VI 서버:일반:G객체", "구조 프레임 인덱스가 범위를 벗어납니다. 이 에러는 케이스, 다층 시퀀스, 또는 이벤트 구조의 프레임에 접근하기 위해 범위를 벗어난 인덱스 값을 사용할 때 발생할 수 있습니다.", "라디오 버튼 컨트롤의 컨트롤에 이 프로퍼티를 사용할 수 없습니다.", "타입 정의 설정의 인스턴스에 이 프로퍼티를 사용하여타입 정의의 원래 복사본으로부터 자동적으로 업데이트할 수 없습니다.", "아주 큰 설명자를 가진 데이터 타입을 생성하려고 시도했습니다.", "VI를 실행 상태에 있지 않은 서브패널에 삽입할 수 없습니다.", "실행 모드에서 LabVIEW는 생성되지 않은 컨트롤 부분에 대해서 프로퍼티를 얻거나 설정할 수 없습니다.", "NI 라이센스 관리자가 초기화되지 않았습니다. 시작≫프로그램≫National Instruments≫NI 라이센스 관리자를 선택하여 컴퓨터에 NI 라이센스 관리자가 설치되었는지 확인합니다.", "유효하지 않은 프로젝트 빌드 참조.", "이 경로의 LabVIEW 파일이 메모리에 이미 존재하거나 또는 메모리에 있는 프로젝트 라이브러리 내에 존재합니다. 이 에러를 해결하려면, 파일의 경로를 열려 있는 어플리케이션 인스턴스에서 아직 LabVIEW 파일을 포함하지 않는 경로로 지정하십시오.", "하위 구획의 최소 또는 최대 크기를 만족하지 못하기 때문에, 분리자 막대를 이 위치로 이동할 수 없습니다. LabVIEW가 분리자 막대를 지정된 위치로 이동하려할 때, 적어도 하나 이상의 구획이 설정된 최소 크기보다 작게 줄어듭니다. 예를 들어, 하나의 수직 분리자 막대를 가진 VI가 있고 왼쪽 구획의 최소 크기가 50인 경우, 분리자 위치 프로퍼티에 10을 연결하면 이 에러가 반환됩니다. 이 에러를 수정하려면, 구획의 최소 크기를 더 작은 값으로 설정하거나, 분리자 위치 프로퍼티에 최소 크기 이상으로 구획을 줄이지 않는 값을 연결하십시오.", "이전의 끌기 트랜잭션이 여전히 대기 상태이기 때문에 끌기가 시작할 수 없습니다.", "이 끌어서 놓기 작업에 요청된 데이터 타입을 제공할 수 없습니다. 이 에러를 수정하려면 이 함수를 호출했을 때 끌기와 놓기 작업이 진행중인지 확인하고 데이터 타입과 끌기 데이터 이름이 끌기와 놓기 작업 도중에 현재 사용 가능한 것과 일치하는지 확인합니다.", "끌기 데이터 원소의 이름 또는 데이터 타입이 내장된 LabVIEW 끌기 데이터 타입과 충돌합니다. 데이터 이름에 접두어 LV_는 사용할 수 없습니다.", "자동 줄바꾸기가 활성화되어 있으면 이 문자열 디스플레이 모드와 함께 이 프로퍼티를 사용할 수 없습니다. 디스플레이 모드를 제로(일반)로 변경하고 이 프로퍼티를 사용하기 위해 자동 줄바꾸기를 비활성화합니다.", "지정된 이름 또는 GUID가 유효하지 않습니다.", "제공자 플러그인이 설치되지 않았거나 훼손되었습니다", "유효한 GUID 생성에 실패하였습니다", "VI가 삽입된 여러 패널을 포함하고 있을때 서브패널 컨트롤의 스크롤 막대를 숨기거나 보일 수 없습니다.", "선택된 빌드는 완료되지 못했습니다.", "다이어그램 비활성화 구조는 기본 프레임을 가지고 있지 않습니다. 이 에러는 기본 프레임 프로퍼티를 다이어그램 비활성화 구조와 함께 사용하려할 때 발생합니다. 이 프로퍼티는 조건적 비활성화 구조와 함께만 사용할 수 있습니다.", "다이어그램 비활성 구조는 조건을 가질 수 없습니다. 이 조건 프로퍼티와 프레임 인덱스 얻기 메소드는 오직 조건적 비활성화 구조와 함께 사용할 수 있습니다.", "조건적 비활성화 구조에 활성 프레임 프로퍼티를 설정할 수 없습니다. 이 에러는 활성 프레임 프로퍼티를 조건적 비활성화 구조와 함께 사용하려할 때 발생합니다. 조건이 활성 프레임을 결정하기 때문에 이 프로퍼티는 조건적인 비활성 구조와 함께 사용될 수 없습니다. 이 프로퍼티는 다이어그램 비활성화 구조와 함께만 사용할 수 있습니다.", "라이센스 체크아웃에 실패하였습니다. 라이센스가 유효하지 않거나 존재하지 않기 때문에 요청된 라이센스를 체크아웃할 수 없습니다.", "1보다 작은 크기의 세마포어는 생성될 수 없습니다.끌기 데이터 타입의 중복된 이름이 끌기 시작 메소드 또는 끌기 시작? 이벤트로 전달되었기 때문에, 끌기를 시작할 수 없습니다. 이 에러를 수정하려면, 끌기 데이터에 사용하는 이름이 메소드 또는 이벤트의 데이터 배열의 각 원소에 유일하도록 하십시오.", "제공된 데이터가 유효하지 않기 때문에, 끌기와 놓기 동작을 시작할 수 없습니다. 이 에러를 수정하려면, 끌기 데이터 배열이 널이 아닌지, 모든 원소가 이름과 데이터 필드를 가지고 있는지 확인하십시오.", "접근하려고 하는 블록다이어그램은 평가판 모드 또는 유효하지 않은 라이센스의 LabVIEW에서 생성된 VI에 포함됩니다. 이 에러를 수정하려면, 해당 VI와 그에 포함된 라이브러리에 대한 유효한 라이센스를 얻어야합니다.", "평가판 모드 또는 유효하지 않은 라이센스의 LabVIEW에서 VI 저장 및 복사를 시도하였습니다. 이 에러를 수정하려면, 해당 VI와 그에 포함된 라이브러리에 대한 유효한 라이센스를 얻어야합니다.", "스코프를 벗어난 VI의 VI 서버 참조를 열려고 시도하였습니다. VI는 subVI로 호출할 수 있는 다른 VI에게만 VI 서버 참조를 열 수 있습니다. 참조가 열린 후에, VI는 일반 상황에서는 참조를 열 수 없는 다른 VI에게도 참조를 반환할 수 있습니다.", "소스 문자 세트의 텍스트를 대상 문자 세트로 변환할 수 없습니다.", "이 subVI의 필수 입력이 연결되어 있지 않습니다. 이 에러를 수정하려면, 필수 입력을 연결합니다.", "블록다이어그램에 로컬 변수가 있기 때문에, subVI는 코드로 대체될 수 없습니다.", "프런트패널 터미널이 루트 다이어그램에 없기 때문에, subVI는 코드로 대체될 수 없습니다. 예를 들어, 이 에러는 프런트패널 터미널이 구조의 안에 있을 때 발생할 수 있습니다.", "경로가 비어있거나 상대 경로입니다. 절대 경로를 반드시 사용해야 합니다.", "지정된 포맷을 부동소수 데이터와 함께 사용할 수 없습니다. 예를 들어, 16진수 표기법은 부동소수에 유효한 포맷이 아닙니다.", "정밀도가 이 포맷에서 허용되는 최대 값보다 큽니다.", "숫자형 정밀도는 음수가 될 수 없습니다.", "아카이브 버전은 현재 LabVIEW 버전보다 더 나중의 것입니다.", "디스크의 새 라이브러리 파일이 원본 라이브러리와 충돌을 일으킬 수 있기 때문에, 프로젝트 라이브러리를 원본 라이브러리와 동일한 폴더에 복사할 수 없습니다. 프로젝트 라이브러리를 복사할 때 반드시 디스크의 다른 위치를 지정해야 합니다.", "파일 이름은 예상된 이름과 일치하지 않습니다. 지정된 파일은 원본 파일과 같은 파일 이름을 가지고 있어야 합니다.", "지정된 서버에 의해 디버그 연결이 거부되었습니다. 어플리케이션 또는 공유 라이브러리당 하나의 디버그 연결만 허용됩니다.", "어플리케이션에서 다운로드할 VI가 없습니다. 연결이 종료되었습니다.", "VI 참조 열기가 더 이상 메모리의 VI들과 파일 이름으로 일치하지 않습니다. VI의 전체 이름이 이제 상위 라이브러리를 포함하기 때문에 파일 이름은 더 이상 유효하지 않습니다. 경로 분리 함수를 사용하여 파일 이름을 문자열로 연결할 수 있지만, 라이브러리에 포함된 VI에는 해당되지 않습니다.", "이전 버전으로 저장할 때 이름 충돌이 있었습니다. 라이브러리의 VI는 라이브러리 이름_VI 이름의 형태로 저장되었습니다. 동일한 이름을 가진 VI가 이미 이 계층구조에 있습니다.", "배열은 적어도 하나의 차원을 가지고 최대 63 차원을 가질 수 있습니다.", "하나 혹은 그 이상의 제목없는 라이브러리가 의존되어 있습니다. 모든 종속 파일의 이름을 만들기 전에는 이 파일을 저장할 수 없습니다.", "하나 혹은 그 이상의 제목없는 의존되어 있습니다. 모든 종속 파일의 이름을 만들기 전에는 이 파일을 저장할 수 없습니다.", "이 라이브러리가 LabVIEW의 이전 버전에서 저장되었습니다. LabVIEW의 현재 버전으로 로드되고 저장되어야 합니다.", "라벨, 캡션, 독립 라벨의 수직 배치를 설정할 수 있습니다.", "LabVIEW 클래스는 LabVIEW의 이 버전에서 XML로 패턴화될 수 없습니다.", "되돌리기를 실패했습니다. 이 아이템이 이 머신에서 다른 내용으로 편집되었습니다. 그 인스턴스만이 되돌려질 수 있습니다.", "라이브러리가 지정된 기능을 지원하지 않습니다. 기능 이름에 공백이 없는지 확인합니다.", "지정된 기능이 이미 있습니다. 기능을 여러번 추가할 수 없습니다.", "지정된 폴더가 라이브러리에 있지 않습니다. 라이브러리 아이템을 라이브러이에 있지 않은 폴더에 추가할 수 없습니다.", "플롯 범례를 자동 크기 조정으로 설정하거나 범례가 하나 이상의 엔트리가 있고 플롯 범례를 수평으로 배치하면 플롯 범례의 폭을 변경할 수 없습니다. 그래프 또는 차트에서 마우스 오른쪽 버튼을 클릭하고 바로 가기 메뉴의 플롯 범례 자동 크기 조정을 선택 해제하여, 크기 자동 조정 기능을 비활성화하고 플롯 범례를 수직으로 정렬했는지 점검합니다.", "SubVI의 블록다이어그램에 함축적인 컨트롤 참조가 있기 때문에 LaVIEW가 subVI를 호출하는 VI로 인라인 할 수 없습니다. 이 에러를 수정하고 subVI를 인라인하려면 함축적인 컨트롤 참조를 제거합니다.", "SubVI의 블록다이어그램에 함축적인 프로퍼티 노드 또는 인보크 노드가 있기 때문에 LaVIEW가 subVI를 호출하는 VI로 인라인 할 수 없습니다. 이 에러를 수정하고 subVI를 인라인하려면 함축적인 프로퍼티 노드 또는 인보크 노드를 제거합니다.", "이동 파일은 더이상 지원되지 않기 때문에 로드할 수 없습니다.", "이동 파일은 그 내용이 유효하지 않거나 손상되어 있기 때문에 로드할 수 없습니다.", "존재하지 않거나 유효하지 않은 데이터를 참조하기 때문에 이동 파일을 로드할 수 없습니다.", "하나의 어플리케이션 인스턴스에서 큐 참조를 얻으면 다른 어플리케이션 인스턴스에서 같은 큐 참조를 사용할 수 없습니다. LabVIEW 어플리케이션 인스턴스 사이의 통신에 큐를 사용할 수 없습니다.", "하나의 어플리케이션 인스턴스에서 알림자 참조를 얻으면 다른 어플리케이션 인스턴스에서 같은 알림자 참조를 사용할 수 없습니다. LabVIEW 어플리케이션 인스턴스 사이의 통신에 알림자를 사용할 수 없습니다.", "같은 이름을 가진 여러 파일이 단일 LLB에 저장될 수 없기 때문에 저장 작업을 실패했습니다. 이 에러를 수정하려면 LLB 대신에 폴더에 저장합니다.", "실행 중인 VI의 인스턴스가 존재할 때 편집하기 위해 라이브러리를 잠금해제할 수 없습니다.", "라이브러리에 에러가 있습니다. 이 작업을 시도하기 전에 에러를 수정하십시오.라이브러리에는 다른 내용으로 편집된 것을 가지고 있습니다. 이 작업을 시도하기 전에 변경사항을 동기화하십시오.", "하나의 어플리케이션 인스턴스에서 사용자 이벤트 참조를 얻으면 다른 어플리케이션 인스턴스에서 같은 사용자 이벤트 참조를 사용할 수 없습니다. LabVIEW 어플리케이션 인스턴스 사이의 통신에 사용자 이벤트를 사용할 수 없습니다.", "블록다이어그램을 포함하지 않고는 적절치 않은 VI를 저장할 수 없습니다.", "재호출 VI의 복제를 저장할 수 없습니다.", "리모트 패널을 저장할 수 없습니다.", "라이브러리 호출 노드 프로세스에서 에러가 발생했습니다. 라이브러리 호출 노드와 DLL에서 호출된 함수 사이에서 호출 형식에 대한 설정이 일치하지 않아서 발생했을 가능성이 높습니다.", "유효하지 않은 개수의 문자열이 문자열 [ ] 프로퍼티로 전달되었습니다. 1개 또는 6개의 문자열을 전달해야 합니다.", "저장힐 타겟 버전이 올바르게 포맷되어 있지 않습니다. 저장하려는 타겟 버전이 다음과 같은 유효한 LabVIEW 버전이어야 합니다: x.x 또는 xx.x, 여기서, x는 숫자입니다. 유효한 버전 목록은 LabVIEW 도움말을 참조하십시오.", "그래프 또는 차트의 플롯 범례가 트리 보기인 경우에는 이 프로퍼티가 적용되지 않습니다.", "하위 VI 호출이 너무 많습니다. 이 에러는 일반적으로 반복에서 이를 중단하는 적절한 터미널 조건이 없을 때 발생합니다.", "타겟 어플리케이션 인스턴스가 현재 삭제되고 있습니다. 어플리케이션 인스턴스에 대한 새 참조를 가져오거나 어플리케이션 인스턴스에서 VI를 로드할 수 없습니다.", "지정된 터미널에서 공유 변수 노드를 생성할 수 없습니다.", "지정한 세마포어가 존재하지 않습니다. LabVIEW는 이 세마포어에 대한 참조를 반환할 수 없습니다. 세마포어 참조 얻기 VI의 발견되지 않으면 생성 입력이 거짓이고, 지정한 이름으로 LabVIEW가 세마포어를 찾을 수 없는 경우에 이 에러가 발생할 수 있습니다.", "지정한 세마포어 참조가 유효하지 않습니다. 이 에러를 수정하려면, 세마포어의 참조가 유효한지 점검합니다.", "LabVIEW가 버퍼되지 않은 모드에서 열린 파일에서 읽기, 쓰기, 찾기 작업을 시도했고, 데이터의 크기가 디스크 섹터 크기의 배수가 아닙니다. 올바른 섹터 크기를 반환하려면 볼륨 정보 얻기 함수를 사용합니다. 섹터 크기와 정렬할 올바른 데이터 크기를 갖고 있지 않은 경우, 필터 데이터로 데이터를 채우고 LabVIEW가 다시 파일을 읽기 전에 필터 데이터를 삭제해야 합니다.", "LabVIEW가 버퍼되지 않은 모드에서 열린 파일에서 데이터를 쓰거나 읽으려고 시도했고, 데이터가 올바르게 정렬되지 않았습니다. LabVIEW는 데이터가 어떻게 정렬되는지를 결정하며, 사용자가 이 정렬 방법을 바꿀 수 없습니다. 이 에러가 발생하는 경우, 버퍼링을 활성화하고 파일을 다시 열어야 합니다.", "VI가 이 프로퍼티를 사용하는 프로젝트에 있어야 합니다.", "크기 0에서는 큐 참조 번호를 얻을 수 없습니다. 입력하는 크기가 양수이거나, 크기 무제한의 경우에는 -1이어야 합니다.", "I/O 서버 타입의 라이센스가 유효하지 않습니다.", "LabVIEW 런타임 엔진은 다형성 VI를 로드할 수 없습니다. 이 에러는 VI가 다형성일 때 독립 어플리케이션에서 발생합니다. 이 에러를 수정하려면, 다형성 VI가 아니라 다형성 VI의 인스턴스를 로드하십시오.", "현재의 LabVIEW 타겟이 컨트롤 VI를 로드할 수 없습니다.", "해당 참조가 유효하지 않습니다. 이 에러의 발생 원인은 참조가 삭제되었기 때문일 수 있습니다.", "LabVIEW가 중복된 참조에 동시에 접근하려고 시도했습니다.", "와이어 타입과 참조의 내부 데이터 타입이 일치하지 않습니다. 이 문제는 타입 캐스트 에러 때문에 발생했을 수 있습니다.", "이 때에 프로젝트 파일을 저장할 수 없습니다. 프로젝트에는 잠긴 제목없는 의존성이 있습니다. 잠금은 제목없는 아이템에 저장할 수 없는 이름을 붙이는 것을 방지합니다.", "LabVIEW 이전 버전에 저장한 묶음 라이브러리는 열 수 없습니다.", "현재 타겟이나 OS와 다른 타겟 또는 OS용으로 만들어진 묶음 라이브러리는 로드할 수 없습니다.", "LabVIEW 런타임 엔진에서 컴파일된 코드가 분리되어있는 파일을 열 수 없습니다. 파일 배급자에게 문의하십시오. 배급자는 LabVIEW 런타임 엔진에서 실행될 수 있도록 반드시 파일에 컴파일된 코드를 포함해야 합니다.", "지정된 경로는 공동의 디렉토리를 공유하지 않습니다. 이 경로는 디렉토리를 공유해야 합니다. 공동의 디렉토리를 공유하는 각 경로 세트에 대해 캐시를 만들어 보십시오.", "컴파일된 객체의 캐시에서 컴파일된 코드를 찾을 수 없습니다. VI가 컴파일된 코드를 따로 저장하도록 표시되었는지, VI가 깨지지 않았는지 확인하십시오. 그런 다음 VI를 컴파일합니다.", ".NET 컨테이너나 ActiveX 컨테이너에서 이 프로퍼티를 사용할 수 없습니다.", "참조에 있는 데이터의 크기를 조정할 수 없습니다. 참조의 데이터와 데이터 값 참조 원소 쓰기 경계 노드에 연결된 데이터의 크기가 맞지 않습니다.", "컴파일된 코드가 이전 버전입니다.", "소스 파일에서 컴파일된 코드를 분리하도록 VI에 표시되어 있지 않습니다.", "컴파일된 객체의 캐시가 손상되었습니다.", "지정된 파일의 의존성 중 유효한 이름이 있는 것을 LabVIEW가 예상하지 못했습니다. 이러한 불일치는 의존성 보고서가 신뢰할 수 없다는 것을 뜻하며, 따라서 링크 정보 읽기 작업이 강제 종료되었습니다.", "RT 타겟에 시작 어플리케이션을 로드할만큼 충분한 메모리가 없습니다.", "SSL이 설정 또는 설치되지 않았거나, 지원되지 않아서 이 OS에서는 SSL을 사용할 수 없습니다.", "바로 가기 메뉴에서 \"붙여넣기\" 옵션이 비활성화되어 있는 대상에 데이터 붙여넣기 작업을 시도했습니다.", "빈 문자열은 유효한 메소드 이름이 아닙니다.", "[VI 참조 열기] 함수는 비동기 참조에 의한 호출 옵션을 재호출 실행 준비 옵션과 함께 사용하도록 지원하지 않습니다. 0x80 및 0x100 옵션 플래그 모두 0x08 옵션 플래그와 충돌합니다. 0x08 플래그는 VI를 VI 실행 메소드와 함께 실행할 때 유용합니다. 0x08 플래그는 비동기화 호출을 수행할 때는 유용하지 않습니다. 이 에러를 수정하려면, 0x08 옵션을 제거하거나 0x80 및 0x100 옵션을 제거하십시오.", "[VI 참조 열기] 함수는 0x08 옵션(재호출 실행 준비)을 비동기 참조에 의한 호출 옵션인 0x80(호출 및 무시 준비) or 0x100(호출 및 수집 준비)과 함께 사용하도록 지원하지 않습니다.", "프런트패널 아이템에 실행 데이터가 없기 때문에 내부 에러가 발생했습니다. VI를 다시 컴파일하면 이 문제가 해결될 수도 있습니다.", "리포트를 저장할 경로가 유효하지 않습니다. 유효한 경로에는 다음 증 어떠한 문자도 포함되서는 안 됩니다: (Windows) < > / | : \" * ? or (OS X/Linux) < > \\ | : \" * ?.", "LabVIEW가 VI 비교 리포트를 생성할 수 없습니다. 지정한 경로에 대해 쓰기 권한이 있는지 확인한 후, 리포트를 다시 생성하십시오.", "LabVIEW가 Microsoft Word 구성요소를 찾을 수 없습니다. Microsoft Word를 올바르게 설치하였는지 확인하십시오.", "LabVIEW가 Microsoft Word 리포트를 생성할 수 없습니다. 리포트 생성을 다시 시도하십시오. 문제가 지속되면, National Instruments 기술 지원에 연락하십시오.", "LabVIEW가 Microsoft Word 리포트를 생성할 수 없습니다. 리포트 생성을 다시 시도하십시오. 문제가 지속되면, National Instruments 기술 지원에 연락하십시오.", "LabVIEW가 Microsoft Word 리포트를 생성할 수 없습니다. Microsoft Word를 올바르게 설치하였는지 확인한 후, 리포트를 다시 생성하십시오.", "LabVIEW가 Microsoft Word 구성요소를 찾을 수 없습니다. Microsoft Word를 올바르게 설치하였는지 확인하십시오.", "OS X 및 Linux에서는 웹 페이지나 일반 텍스트 리포트만을 생성할 수 있습니다.", "%d의 위치에 있는 컨트롤 인덱스가 유효하지 않습니다.", "LabVIEW는 %d의 위치에 있는 입력 데이터 타입을 컨트롤 데이터 타입으로 변경할 수 없습니다.", "이 컨트롤은 블록다이어그램에서 터미널을 가지고 있어야 합니다.", "배리언트 또는 LabVIEW 클래스 라이브러리 파일(.lvclass)를 이 함수에 연결하는 경우, 같은 어플리케이션 인스턴스에 있는 VI에서 함수를 호출해야 합니다.", "사용자 컨트롤을 직접 서브패널에 삽입할 수 없습니다. 대신 프런트패널에 사용자 컨트롤이 있는 VI를 사용하십시오.", "선택된 디바이스가 유효하지 않습니다. 현재 선택된 디바이스 인덱스가 유효하지 않습니다. 유효하지 않은 사운드 드라이버로 인해 이 에러가 발생할 수 있습니다.", "유효하지 않은 사운드 태스크 참조 번호. 사용할 사운드 드라이버가 없거나 주어진 GUID가 유효한 DirectSound 디바이스 ID가 아닙니다.", "사운드 디바이스가 사용 중에 있습니다. 다른 어플리케이션이 현재 디바이스를 사용하고 있습니다. 이 어플리케이션의 우선순위 레벨을 높이면 이 문제가 해결될 수 있습니다.", "사운드 드라이버 또는 카드가 지정된 설정과 호환되지 않습니다. 입력된 파라미터가 하드웨어 및 드라이버의 지원 범위 내에 있는지 확인합니다. 사운드 출력 설정 VI를 사용하는 동안 이 에러가 발생했다면, 더 자세한 정보는 ni.com에서 기술지원 데이터베이스를 참조하십시오.", "파일 재생 장치에 쓸 수 없습니다. 파일이 재생되는 동안 어플리케이션이 파일에 쓰려고 시도하였습니다. 이 에러 코드는 현재 LVSound 라이브러리에 의해 보고되지 않습니다.", "사운드 파일을 찾을 수 없습니다. 지정된 사운드 파일을 찾을 수 없습니다.", "실행하기 위해서 DirectX 8.0 또는 상위 버전이 필요합니다. 이 에러를 수정하려면 http://www.microsoft.com/downloads에서 최신 DirectX 버전을 설치하십시오.", "사운드 포맷을 인식할 수 없습니다. 이 파일의 사운드 포맷을 인식할 수 없습니다. 파일이 손상되었을 수도 있습니다.", "사운드 포맷을 지원하지 않습니다. 지정된 웨이브 포맷을 지원하지 않습니다. 하드웨어, 드라이버, 또는 양쪽 모두의 한계일 수도 있습니다.", "버퍼 언더플로우가 발생하였습니다. 어플리케이션이 데이터를 쓰는 속도가 빠르지 않아 버퍼 언더플로우가 발생하였습니다.", "덮어쓰기 에러. 어플리케이션이 버퍼에서 데이터를 읽는 속도가 빠르지 않아 덮어쓰기 에러가 발생하였습니다.", "수행이 완료되기 전에 타임아웃이 발생하였습니다. 어플리케이션이 성공적으로 상호 배제를 얻을 수 없었기 때문에 타임아웃 에러가 발생하였습니다.", "활성화된 태스크 없이 이 작업을 수행할 수 없습니다. 이 태스크가 활성화되어 있는지 확인하고 다시 시도하십시오. 입력 버퍼가 오버플로우 상태이면, 입력 태스크가 실행을 정지할 수 있습니다. 데이터를 충분히 빨리 읽지 않을 때 오버플로우가 발생합니다.", "일반 프로젝트 에러.", "이 이름의 아이템이 프로젝트에 이미 존재합니다.", "이 경로의 아이템이 프로젝트에 이미 존재합니다.", "이 아이템을 추가하면 다른 아이템과 충돌할 수 있습니다.", "프로젝트 아이템을 찾을 수 없습니다.", "아이템 타입이 타겟 타입과 호환되지 않습니다.", "프로젝트 라이브러리에 묶음 라이브러리를 추가할 수 없습니다.", "컨트롤러의 글로벌 시간이 변경되었고, NI 스캔 엔진의 반복 주기가 영향을 받을 수 있습니다. IEEE-1588 또는 GPS와 같은 타이밍 소스가 컨트롤러의 글로벌 시간 값을 수정했습니다. 이때 임시적인 위상 이동이 있을 수 있고, 그런 경우 NI 스캔 엔진 변수의 1회 반복 업데이트 주기가 변경됩니다."] ("String Data"), index=w113) -> (element=w106:string)
          n45 = Concatenate Strings(w110, w105, "error", w107, w108, w105, w106, w105) -> (w104:string)
          n46 = call "에러창"() -> ("확인"=w126:bool)  [unwired: 10 in, 1 out]
          n47 = call <vilib>:"Application Directory.vi"() -> ("Application Directory"=w115:path)
          n48 = Path To String(path=w115) -> (string=w117:string)
          n49 = case shown="참" w126 {
            tunnel: w121 -> [_ w149]
            tunnel: w120 -> [_ w148]
            tunnel: w104 -> [_ w128]
            frame False {
            }
            frame True {
              n50 = call "e-mail을 입력해 주세요."() -> ("E-Mail"=w146:string)  [unwired: 17 in, 2 out]
              n51 = call <vilib>:"Application Directory.vi"() -> ("Application Directory"=w138:path)
              n52 = Path To String(path=w138) -> (string=w136:string)
              n53 = Concatenate Strings(w136, "\\data\\name.ini" ("문자열")) -> (w137:string)
              n54 = String To Path(string=w137) -> (path=w135:path)
              n55 = Concatenate Strings(w149, w148, "e-mail :" ("문자열"), w146) -> (w134:string)
              n56 = call <vilib>:"Open Config Data.vi"("configuration file path"=w135) -> ("error out"=w143:errorcluster, "refnum"=w144:T3)  [unwired: 8 in, 1 out]
              n57 = call-poly <vilib>:"Read Key.vi"("section"="name", "error in (no error)"=w143, "key"="name", "refnum"=w144) -> ("error out"=w142:errorcluster, "value"=w131:string, "refnum out"=w141:T3)  [unwired: 4 in, 1 out]
              n58 = Concatenate Strings(w134, "\r", "사용자닉네임 :", w131) -> (w130:string)
              n59 = call <vilib>:"Close Config Data.vi"("error in (no error)"=w142, "refnum"=w141) -> ()  [unwired: 8 in, 2 out]
              n60 = Concatenate Strings(w130, "\r", w128) -> (w127:string)
              n61 = call "에러리포트"("Message"=w127) -> ()  [unwired: 10 in, 1 out]
            }
          }
          n62 = Concatenate Strings(w117, "\\data\\errorlog.pbfs" ("문자열")) -> (w118:string)
          n63 = String To Path(string=w118) -> (path=w119:path)
          n64 = Write to Text File(file (use dialog)=w119, text=w104) -> (refnum out=w114:refnum<file>)  [unwired: 2 in, 2 out]
          n65 = Close File(refnum=w114) -> ()  [unwired: 1 in, 2 out]
        }
      }
    }
    frame #2 {
      w154 = "/airport_data/airport_data.txt"  # remote read path
      w155 = "93.188.160.178"  # host
      # "gom20726!"
      # "01050034508"
      # "tkddn4508@gmail.com"
      # "user"
      # "password"
      # "공항데이터 업데이트"
      n66 = call <vilib>:"FTP Get Buffer.vi"("password"=w152, "user"=w151, "remote path"=w154, "host"=w155) -> ("error out"=w150:errorcluster, "data"=w153:string)  [unwired: 5 in, 1 out]
      n67 = call <vilib>:"Clear Errors.vi"("error in (no error)"=w150) -> ()  [unwired: 5 in, 2 out]
      n68 = case shown="에러 없음" w150 {
        tunnel: w153 -> [w157 _]
        frame No Error {
          # "에러 유무"
          n69 = flat-sequence {
            tunnel: w157 -> [w159]
            tunnel: [w159] -> w156
            tunnel: w156 -> [w161]
            frame #0 {
              # "업데이트 알림"
              n70 = local write "정보출력"("airport_data 업데이트가 존재 합니다. ") -> ()
            }
            frame #1 {
              # "data update"
              # "공항데이터 업데이트"
              n71 = call <vilib>:"Application Directory.vi"() -> ("Application Directory"=w177:path)
              n72 = Path To String(path=w177) -> (string=w175:string)
              n73 = Match Pattern(string=w161, regular expression="<update>" ("정규식")) -> (after substring=w172:string)  [unwired: 1 in, 3 out]
              n74 = Concatenate Strings(w175, "\\data\\airport_data" ("문자열")) -> (w174:string)
              n75 = Match Pattern(string=w172, regular expression="</update>" ("정규식")) -> (before substring=w166:string)  [unwired: 1 in, 3 out]
              n76 = String To Path(string=w174) -> (path=w160:path)
              n77 = Read from Text File(file (use dialog)=w160) -> (text=w167:string)  [unwired: 3 in, 3 out]
              n78 = Match Pattern(string=w167, regular expression="<update>" ("정규식")) -> (after substring=w169:string)  [unwired: 1 in, 3 out]
              n79 = Match Pattern(string=w169, regular expression="</update>" ("정규식")) -> (before substring=w165:string)  [unwired: 1 in, 3 out]
              n80 = global write "airport경로.vi" "경로"(w160) -> ()
              n81 = call <vilib>:"Trim Whitespace.vi"("string"=w166) -> ("trimmed string"=w163:string)  [unwired: 1 in]
              n82 = call <vilib>:"Trim Whitespace.vi"("string"=w165) -> ("trimmed string"=w164:string)  [unwired: 1 in]
              n83 = Equal?(x=w163, y=w164) -> (x = y?=w162:bool)
              n84 = case shown="거짓" w162 {
                tunnel: w160 -> [w186 _]
                tunnel: w161 -> [w180 _]
                tunnel: w164 -> [w179 _]
                tunnel: w163 -> [w178 _]
                frame False {
                  n85 = Write to Text File(file (use dialog)=w186, text=w180) -> ()  [unwired: 2 in, 3 out]
                  n86 = Concatenate Strings(w178, "update success" ("문자열"), "\r", "기존 버전은", w179, "입니다." ("문자열")) -> (w181:string)
                  n87 = call "?"("Message"=w181) -> ()  [unwired: 9 in, 2 out]
                }
                frame True {
                }
              }
            }
          }
        }
        frame Error {
        }
      }
    }
    frame #3 {
      w189 = 128  # call and forget
      # "route finder 호출"
      n88 = disable-structure shown="활성화" {
        frame Disabled {
          w206 = 128  # call and forget
          n89 = Current VI's Path() -> (path=w197:path)
          n90 = Build Path(base path=w197, name or relative path="SUB\\route.vi" ("이름 또는 상대 경로")) -> (appended path=w199:path)
          n91 = Open VI Reference(type specifier VI Refnum (for type only)=refnum<vi> refnum, vi path=w199, options=w206) -> (vi reference=w201:refnum<vi>, error out=w204:errorcluster)  [unwired: 3 in]
          n92 = call-by-ref "Start Asynchronous Call"(reference=w201, error in=w204) -> (reference out=w200:refnum<vi>, error out=w203:errorcluster)  [unwired: 12 in]
          n93 = Close Reference(reference=w200, error in (no error)=w203) -> (error out=w202:errorcluster)
          n94 = call <vilib>:"Simple Error Handler.vi"("error in (no error)"=w202) -> ()  [unwired: 4 in, 5 out]
        }
        frame Enabled {
        }
      }
      n95 = vi-ref "route.vi"() -> (w188:refnum<vi>)
      n96 = property class="VI"(reference=w188) -> (error out=w194:errorcluster, "Path"=w187:path)  [unwired: 1 in, 1 out]
      n97 = Open VI Reference(type specifier VI Refnum (for type only)=refnum<vi> refnum, vi path=w187, options=w189, error in (no error)=w194) -> (vi reference=w195:refnum<vi>, error out=w191:errorcluster)  [unwired: 2 in]
      n98 = call-by-ref "Start Asynchronous Call"(reference=w195, error in=w191) -> (reference out=w196:refnum<vi>, error out=w192:errorcluster)  [unwired: 12 in]
      n99 = Close Reference(reference=w196, error in (no error)=w192) -> (error out=w193:errorcluster)
      n100 = call <vilib>:"Simple Error Handler.vi"("error in (no error)"=w193) -> ()  [unwired: 4 in, 5 out]
    }
    frame #4 {
      # "updater 종료"
      n101 = while {
        tunnel: [w209] -> w207
        stop <- TRUE stop-if-true
        n102 = control-ref of="This VI"() -> (w209:refnum<vi>)
      }
      n103 = invoke class="VI" method="FP.Close"(reference=w207) -> ()  [unwired: 2 in, 3 out]
    }
  }
